vi "test check_login.vi"() -> ()   [LabVIEW 2023]
uses:
  Database.lvlib
panel:
  in  "db password":string="blueberries"
  in  "db username":string="amironov"
  out "error out":errorcluster
  in  "port":i32=3306
  in  "host":string="localhost"
  in  "password":string="carriker"
  in  "username":string="root"
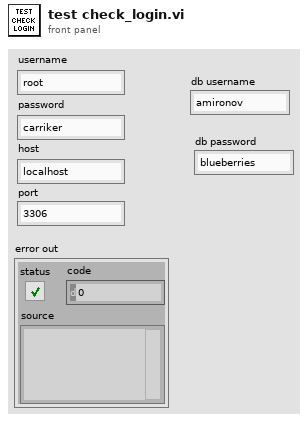
[diagram p1: front panel]
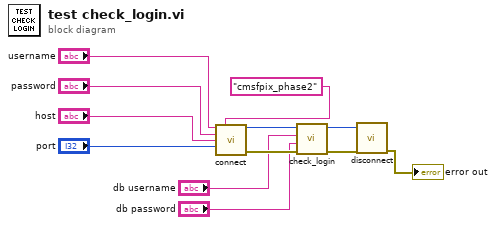
[diagram p0: block diagram]
diagram:
  n1 = call "connect.vi"("username"="username", "schema"="cmsfpix_phase2" ("Schema"), "password"="password", "host"="host", "port"="port") -> ("DB Session ID"=w7:i32, "error out"=w6:errorcluster)  [unwired: 9 in]
  n2 = call "check_login.vi"("error in (no error)"=w6, "password"="db password", "username"="db username", "DB Session ID"=w7) -> ("error out"=w2:errorcluster, "DB Session ID out"=w3:i32)  [unwired: 6 in]
  n3 = call "disconnect.vi"("DB Session ID"=w3, "error in (no error)"=w2) -> ("error out"=→"error out":errorcluster)  [unwired: 13 in]
